vi "MFC.vi"() -> ()   [LabVIEW 2013]
uses:
  <vilib>/NI/Current Value Table/Read tags into grouped data.vi
  <vilib>/NI/Current Value Table/Read Index Set.vi
  <vilib>/NI/Current Value Table/DataTypes/Double_Read Index Set.vi
  <vilib>/NI/Current Value Table/DataTypes/Array of String_Read Index Set.vi
  <vilib>/NI/Current Value Table/DataTypes/Array of Boolean_Read Index Set.vi
  <vilib>/NI/Current Value Table/DataTypes/Array of Single_Read Index Set.vi
  <vilib>/NI/Current Value Table/DataTypes/Array of Double_Read Index Set.vi
  <vilib>/NI/Current Value Table/DataTypes/Array of I8_Read Index Set.vi
  <vilib>/NI/Current Value Table/DataTypes/Array of I16_Read Index Set.vi
  <vilib>/NI/Current Value Table/DataTypes/Array of I32_Read Index Set.vi
  <vilib>/NI/Current Value Table/DataTypes/Array of I64_Read Index Set.vi
  <vilib>/NI/Current Value Table/DataTypes/Array of U64_Read Index Set.vi
  <vilib>/NI/Current Value Table/DataTypes/Array of U32_Read Index Set.vi
  <vilib>/NI/Current Value Table/DataTypes/Array of U16_Read Index Set.vi
  <vilib>/NI/Current Value Table/DataTypes/Array of U8_Read Index Set.vi
  <vilib>/NI/Current Value Table/DataTypes/Boolean_Read Index Set.vi
  <vilib>/NI/Current Value Table/DataTypes/String_Read Index Set.vi
  <vilib>/NI/Current Value Table/DataTypes/U8_Read Index Set.vi
  <vilib>/NI/Current Value Table/DataTypes/U16_Read Index Set.vi
  <vilib>/NI/Current Value Table/DataTypes/U32_Read Index Set.vi
  <vilib>/NI/Current Value Table/DataTypes/U64_Read Index Set.vi
  <vilib>/NI/Current Value Table/DataTypes/I8_Read Index Set.vi
  <vilib>/NI/Current Value Table/DataTypes/I16_Read Index Set.vi
  <vilib>/NI/Current Value Table/DataTypes/I32_Read Index Set.vi
  <vilib>/NI/Current Value Table/DataTypes/I64_Read Index Set.vi
  <vilib>/NI/Current Value Table/DataTypes/Single_Read Index Set.vi
  <vilib>/NI/Current Value Table/FGVs/Group Memory.vi
  <vilib>/NI/Current Value Table/Memory Block.vi
  <vilib>/NI/Current Value Table/DataTypes/Double_Memory Block.vi
  <vilib>/NI/Current Value Table/DataTypes/Array of String_Memory Block.vi
  <vilib>/NI/Current Value Table/DataTypes/Array of Boolean_Memory Block.vi
  <vilib>/NI/Current Value Table/DataTypes/Array of Single_Memory Block.vi
  <vilib>/NI/Current Value Table/DataTypes/Array of Double_Memory Block.vi
  <vilib>/NI/Current Value Table/DataTypes/Array of I8_Memory Block.vi
  <vilib>/NI/Current Value Table/DataTypes/Array of I16_Memory Block.vi
  <vilib>/NI/Current Value Table/DataTypes/Array of I32_Memory Block.vi
  <vilib>/NI/Current Value Table/DataTypes/Array of I64_Memory Block.vi
  <vilib>/NI/Current Value Table/DataTypes/Array of U64_Memory Block.vi
  <vilib>/NI/Current Value Table/DataTypes/Array of U32_Memory Block.vi
  <vilib>/NI/Current Value Table/DataTypes/Array of U16_Memory Block.vi
  <vilib>/NI/Current Value Table/DataTypes/Array of U8_Memory Block.vi
  <vilib>/NI/Current Value Table/DataTypes/Boolean_Memory Block.vi
  <vilib>/NI/Current Value Table/DataTypes/String_Memory Block.vi
  <vilib>/NI/Current Value Table/DataTypes/U8_Memory Block.vi
  <vilib>/NI/Current Value Table/DataTypes/U16_Memory Block.vi
  <vilib>/NI/Current Value Table/DataTypes/U32_Memory Block.vi
  <vilib>/NI/Current Value Table/DataTypes/U64_Memory Block.vi
  <vilib>/NI/Current Value Table/DataTypes/I8_Memory Block.vi
  <vilib>/NI/Current Value Table/DataTypes/I16_Memory Block.vi
  <vilib>/NI/Current Value Table/DataTypes/I32_Memory Block.vi
  <vilib>/NI/Current Value Table/DataTypes/I64_Memory Block.vi
  <vilib>/NI/Current Value Table/DataTypes/Single_Memory Block.vi
  <vilib>/NI/Current Value Table/Current Value Table.lvlib
panel:
  out "error out":errorcluster
  in  "XV-131":bool
  out "PI-131":dbl format="%.1f"
  in  "N2CO2Switch 3":bool
  in  "N2CO2Switch":bool
  out "MFC-102 PV":dbl
  in  "MFC-102":dbl
  in  "XV-102":bool
  in  "XV-111":bool
  in  "MFC-111":dbl
  in  "MFC-101":dbl
  out "MFC-111-PV":dbl format="%.4f"
  in  "XV-101":bool
  out "MFC-101-PV":dbl format="%.4f"
  in  "XV-121":bool
  out "MFC-202-PV":dbl
  in  "MFC-202":dbl
  in  "N2CO2Switch 2":bool
  in  "XV-200":bool
  out "MFC-201-PV":dbl
  in  "MFC-201":dbl
  # "Feeder"
  # "Argon"
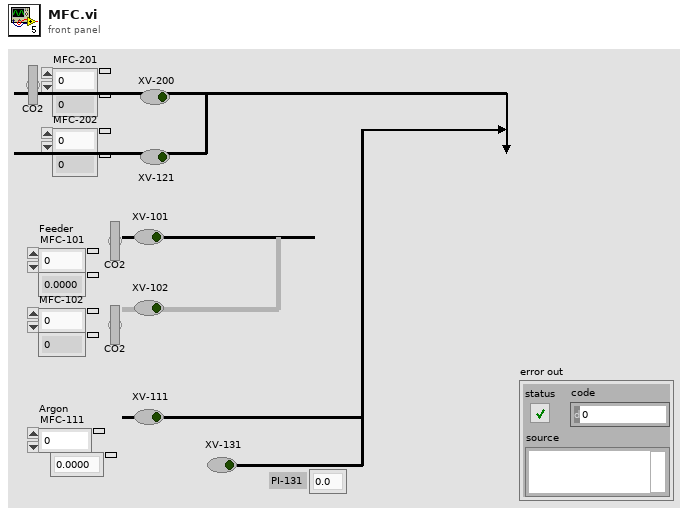
[diagram p1: front panel]
types:
  T1 = typedef "Current Value Table.lvlib/Group Data.ctl" = cluster{"Double":dbl[], "Single":sgl[], "I64":i64[], "I32":i32[], "I16":i16[], "I8":i8[], "U64":u64[], "U32":u32[], "U16":u16[], "U8":u8[], "String":string[], "Boolean":bool[], "Array of U8":cluster{"U8 Array":u8[]}[], "Array of U16":cluster{"U16 Array":u16[]}[], "Array of U32":cluster{"U32 Array":u32[]}[], "Array of U64":cluster{"U64 Array":u64[]}[], "Array of I64":cluster{"I64 Array":i64[]}[], "Array of I32":cluster{"I32 Array":i32[]}[], "Array of I16":cluster{"I16 Array":i16[]}[], "Array of I8":cluster{"I8 Array":i8[]}[], "Array of Double":cluster{"DBL Array":dbl[]}[], "Array of Single":cluster{"SGL Array":sgl[]}[], "Array of Boolean":cluster{"Boolean Array":bool[]}[], "Array of String":cluster{"String Array":string[]}[]}
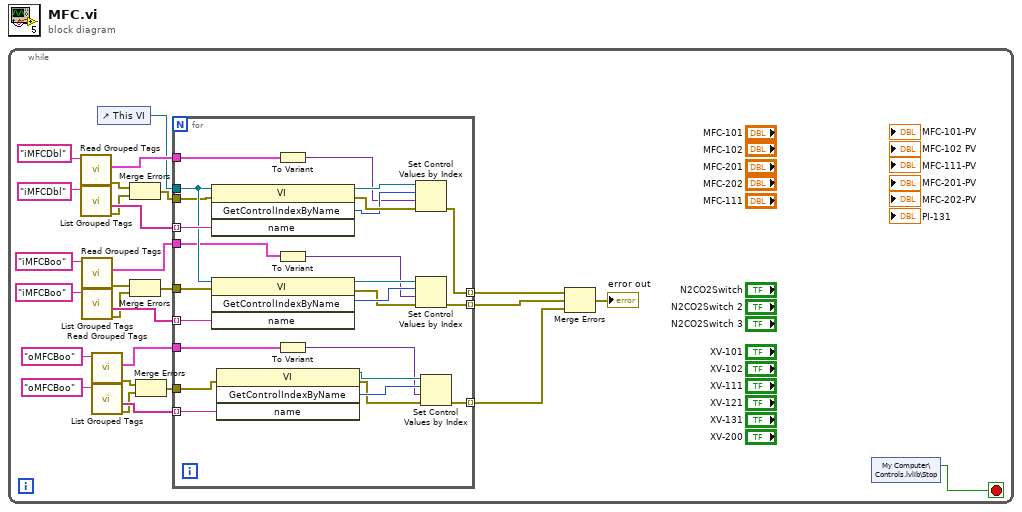
[diagram p0: block diagram]
diagram:
  n1 = while {
    stop <- w10 stop-if-true
    n2 = call <vilib>:"Read Grouped Tags.vi"("Group"="iMFCDbl") -> ("error out"=w9:errorcluster, "Data"=w27:T1)  [unwired: 9 in]
    n3 = call <vilib>:"List Grouped Tags.vi"("Group"="iMFCDbl") -> ("error out"=w8:errorcluster, "Tags Out"=w26:string[])  [unwired: 9 in]
    n4 = call <vilib>:"Read Grouped Tags.vi"("Group"="iMFCBoo") -> ("error out"=w6:errorcluster, "Data"=w22:T1)  [unwired: 9 in]
    n5 = call <vilib>:"List Grouped Tags.vi"("Group"="iMFCBoo") -> ("error out"=w5:errorcluster, "Tags Out"=w21:string[])  [unwired: 9 in]
    n6 = call <vilib>:"Read Grouped Tags.vi"("Group"="oMFCBoo") -> ("error out"=w3:errorcluster, "Data"=w18:T1)  [unwired: 9 in]
    n7 = call <vilib>:"List Grouped Tags.vi"("Group"="oMFCBoo") -> ("error out"=w2:errorcluster, "Tags Out"=w17:string[])  [unwired: 9 in]
    n8 = control-ref of="This VI"() -> (w25:refnum<vi>)
    n9 = Merge Errors(w9, w8) -> (w7:errorcluster)
    n10 = Merge Errors(w6, w5) -> (w4:errorcluster)
    n11 = Merge Errors(w3, w2) -> (w1:errorcluster)
    n12 = for {
      tunnel: w27 -> [w50]
      tunnel: w26 -> [w49] mode=indexing
      tunnel: w25 -> [w43]
      tunnel: w22 -> [w42]
      tunnel: w21 -> [w40] mode=indexing
      tunnel: w18 -> [w35]
      tunnel: w17 -> [w34] mode=indexing
      tunnel: [w33] -> w14 mode=indexing
      tunnel: [w32] -> w13 mode=indexing
      tunnel: [w31] -> w12 mode=indexing
      tunnel: w7 -> [w30]
      tunnel: w4 -> [w29]
      tunnel: w1 -> [w28]
      n13 = invoke class="VI" method="GetControlIndexByName"(reference=w43, error in=w30, "name"=w49) -> (reference out=w52:refnum<vi>, error out=w51:errorcluster, "GetControlIndexByName"=w48:i32)  [unwired: 1 in, 1 out]
      n14 = invoke class="VI" method="GetControlIndexByName"(reference=w43, error in=w29, "name"=w40) -> (reference out=w46:refnum<vi>, error out=w44:errorcluster, "GetControlIndexByName"=w45:i32)  [unwired: 1 in, 1 out]
      n15 = invoke class="VI" method="GetControlIndexByName"(error in=w28, "name"=w34) -> (reference out=w39:refnum<vi>, error out=w37:errorcluster, "GetControlIndexByName"=w38:i32)  [unwired: 2 in, 1 out]
      n16 = To Variant(anything=w50) -> (Variant=w47:variant)
      n17 = To Variant(anything=w42) -> (Variant=w41:variant)
      n18 = To Variant(anything=w35) -> (Variant=w36:variant)
      n19 = Set Control Values by Index(0:w52, 1:w48, 2:w47, 3:w51) -> (11:w33:errorcluster)
      n20 = Set Control Values by Index(0:w46, 1:w45, 2:w41, 3:w44) -> (11:w32:errorcluster)
      n21 = Set Control Values by Index(0:w39, 1:w38, 2:w36, 3:w37) -> (11:w31:errorcluster)
    }
    n22 = Merge Errors(w14, w13, w12) -> (→"error out":errorcluster)
    n23 = shared-variable "My Computer\\Controls.lvlib\\Stop"() -> (w10:bool)  [unwired: 1 in, 1 out]
  }
